vi "Write.EngineData.vi"(8 "error in":errorcluster, 11 "Write in":refnum<class "Write.lvclass">) -> (0 "error out":errorcluster, 3 "Write out":refnum<class "Write.lvclass">)   [LabVIEW 2024, in "VS Plugin Data Access Engine.lvlib" / "Write.lvclass"]
uses:
  Write.lvclass
  Write.lvclass/Write.ctl
  VS Engine Abstraction/VS Engine Interface/VS Engine Interface.lvclass
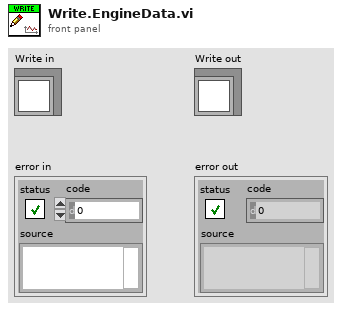
[diagram p1: front panel]
types:
  T1 = typedef "Custom Device API.lvlib/Data Reference.ctl" = i32
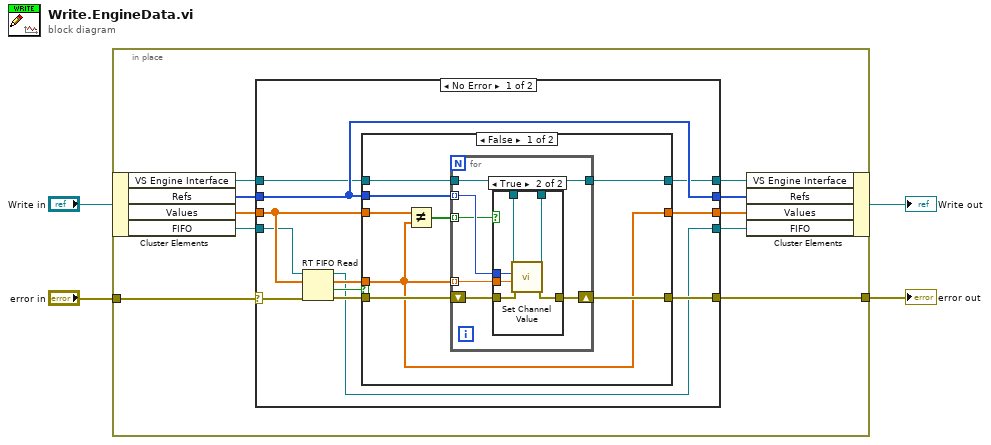
[diagram p0: block diagram]
diagram:
  n1 = in-place {
    in-place-border: [w14] -> w3
    in-place-border: "error in" -> [w13]
    n2 = in-place-cluster #1("Write in") -> ("VS Engine Interface"=w6:refnum<class "VS Engine Interface.lvclass">, "Refs"=w12:T1[], "Values"=w11:dbl[], "FIFO"=w8:refnum<k33>)
    n3 = case shown="No Error" w13 {
      selector: w13 -> [w24 w57]
      tunnel: [w26 w57] -> w14
      tunnel: [w20 w56] -> w10
      tunnel: w12 -> [w19 w55]
      tunnel: w11 -> [w21 w56]
      tunnel: [w19 w55] -> w9
      tunnel: w8 -> [w18 w54]
      tunnel: [w17 w54] -> w7
      tunnel: w6 -> [w16 w53]
      tunnel: [w15 w53] -> w5
      frame No Error {
        n4 = RT FIFO Read(0:w18, 1:w21, 3:w24) -> (8:w17:refnum<k33>, 9:w23:dbl[], 10:w22:bool, 11:w25:errorcluster)  [unwired: 1 in, 1 out]
        n5 = case shown="False" w22 {
          tunnel: w25 -> [w34 w52]
          tunnel: w23 -> [w29 _]
          tunnel: [w33 w52] -> w26
          tunnel: [w29 w51] -> w20
          tunnel: w19 -> [w32 _]
          tunnel: w21 -> [w30 w51]
          tunnel: w16 -> [w28 w50]
          tunnel: [w27 w50] -> w15
          frame False {
            n6 = Not Equal?(x=w30, y=w29) -> (x != y?=w31:bool[])
            n7 = for {
              shift-right: [w41] -> w33
              shift-left: w34 -> [w40]
              tunnel: w31 -> [w37] mode=indexing
              tunnel: w29 -> [w39] mode=indexing
              tunnel: w32 -> [w38] mode=indexing
              tunnel: w28 -> [w36]
              tunnel: [w35] -> w27
              n8 = case shown="True" w37 {
                tunnel: w39 -> [_ w46]
                tunnel: [w43 w48] -> w41
                tunnel: w40 -> [w43 w49]
                tunnel: w38 -> [_ w47]
                tunnel: w36 -> [w42 w45]
                tunnel: [w42 w44] -> w35
                frame False {
                }
                frame True {
                  n9 = call-dynamic "Set Channel Value.vi"("error in"=w49, "Value"=w46, "Data Reference in"=w47, "VS Engine Interface in"=w45) -> ("error out"=w48:errorcluster, "VS Engine Interface out"=w44:refnum<class "VS Engine Interface.lvclass">)  [unwired: 6 in]
                }
              }
            }
          }
          frame True {
          }
        }
      }
      frame Error {
      }
    }
    n10 = in-place-cluster #1("VS Engine Interface"=w5, "Refs"=w9, "Values"=w10, "FIFO"=w7) -> (→"Write out":refnum<class "Write.lvclass">)
  }
  "error out" <- w3
